vi "CF_TC_to_DSC.vi"(0 "description, string":refnum<k21>="ni.var.psp://housesoftheholy/Leiden CF900/CF_TC_description", 1 "dbl var":refnum<k21>[](array[refnum])=["ni.var.psp://housesoftheholy/Leiden CF900/Leiden CF TC/CF TC R0", "ni.var.psp://housesoftheholy/Leiden CF900/Leiden CF TC/CF TC R1", "ni.var.psp://housesoftheholy/Leiden CF900/Leiden CF TC/CF TC R2", "ni.var.psp://housesoftheholy/Leiden CF900/Leiden CF TC/CF TC R3", "ni.var.psp://housesoftheholy/Leiden CF900/Leiden CF TC/CF TC R4", "ni.var.psp://housesoftheholy/Leiden CF900/Leiden CF TC/CF TC R5", "ni.var.psp://housesoftheholy/Leiden CF900/Leiden CF TC/CF TC R6", "ni.var.psp://housesoftheholy/Leiden CF900/Leiden CF TC/CF TC R7", "ni.var.psp://housesoftheholy/Leiden CF900/Leiden CF TC/CF TC T0", "ni.var.psp://housesoftheholy/Leiden CF900/Leiden CF TC/CF TC T1", "ni.var.psp://housesoftheholy/Leiden CF900/Leiden CF TC/CF TC T2", "ni.var.psp://housesoftheholy/Leiden CF900/Leiden CF TC/CF TC T3", "ni.var.psp://housesoftheholy/Leiden CF900/Leiden CF TC/CF TC T4", "ni.var.psp://housesoftheholy/Leiden CF900/Leiden CF TC/CF TC T5", "ni.var.psp://housesoftheholy/Leiden CF900/Leiden CF TC/CF TC T6", "ni.var.psp://housesoftheholy/Leiden CF900/Leiden CF TC/CF TC T7", "ni.var.psp://housesoftheholy/Leiden CF900/Leiden CF TC/CF TC I0", "ni.var.psp://housesoftheholy/Leiden CF900/Leiden CF TC/CF TC I1", "ni.var.psp://housesoftheholy/Leiden CF900/Leiden CF TC/CF TC I2", "ni.var.psp://housesoftheholy/Leiden CF900/Leiden CF TC/CF TC I3"], 2 "dbl":dbl[](array[numeric]), 5 "String In":string, 7 "calibration string":refnum<k21>="ni.var.psp://housesoftheholy/Leiden CF900/CF_TC_calibration", 9 "String In 2":string, 11 "error in (no error)":errorcluster) -> (15 "error out":errorcluster)   [LabVIEW 2016]
panel:
  # "CF TC to DSC"
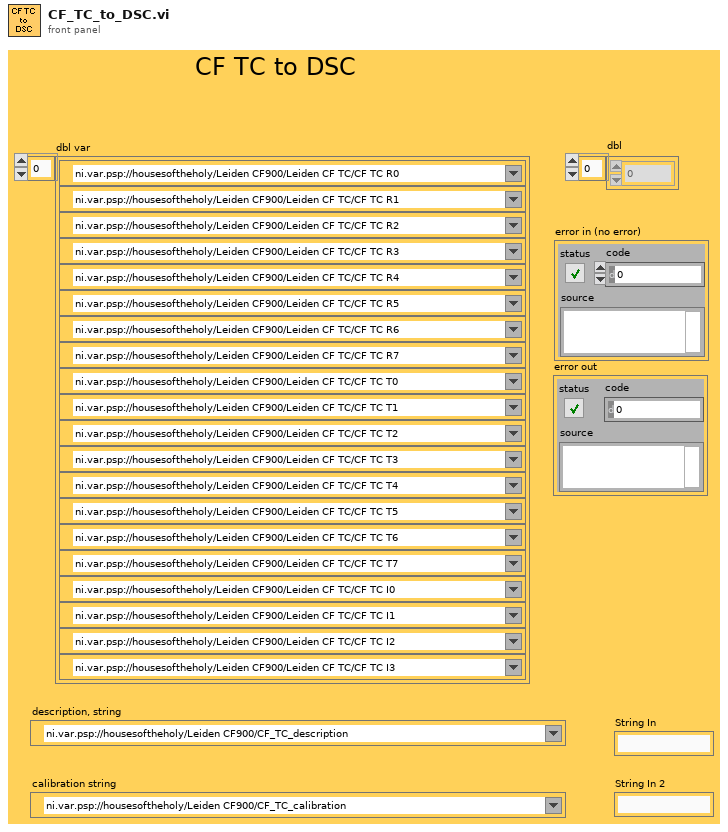
[diagram p1: front panel]
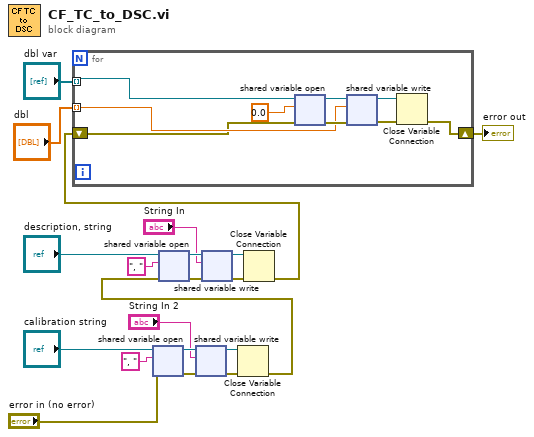
[diagram p0: block diagram]
diagram:
  n1 = shared-variable-open("calibration string", "error in (no error)", ", " ("string")) -> (w12:refnum<k21>, w11:errorcluster)  [unwired: 1 in]
  n2 = shared-variable-write(w12, w11, "String In 2") -> (w13:refnum<k21>, w10:errorcluster)
  n3 = Close Variable Connection(8:w10, 11:w13) -> (0:w4:errorcluster)
  n4 = shared-variable-open("description, string", w4, ", " ("string")) -> (w17:refnum<k21>, w16:errorcluster)  [unwired: 1 in]
  n5 = shared-variable-write(w17, w16, "String In") -> (w18:refnum<k21>, w15:errorcluster)
  n6 = Close Variable Connection(8:w15, 11:w18) -> (0:w3:errorcluster)
  n7 = for {
    tunnel: "dbl var" -> [w24] mode=indexing
    tunnel: "dbl" -> [w23] mode=indexing
    shift-right: [w21] -> w2
    shift-left: w3 -> [w22]
    n8 = shared-variable-open(w24, w22, 0.0) -> (w29:refnum<k21>, w25:errorcluster)  [unwired: 1 in]
    n9 = shared-variable-write(w29, w25, w23) -> (w28:refnum<k21>, w26:errorcluster)
    n10 = Close Variable Connection(8:w26, 11:w28) -> (0:w21:errorcluster)
  }
  "error out" <- w2
